vi "dfd_FXP Casting.vi"   [LabVIEW 2017, in "NI_DigFilter_FXP.lvlib"]
uses:
  <vilib>/addons/Digital Filter Design/NI_DigFilter_FXP.lvlib
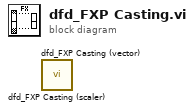
[diagram p0: block diagram]
diagram:
  n1 = call <vilib>:"dfd_FXP Casting (scaler).vi"() -> ()  [unwired: 7 in, 3 out]
  n2 = call <vilib>:"dfd_FXP Casting (vector).vi"() -> ()  [unwired: 7 in, 3 out]
